vi "Start.vi"(11 "Core Actor in":refnum<class "Core Actor.lvclass">) -> (3 "Core Actor out":refnum<class "Core Actor.lvclass">)   [LabVIEW 2025, in "jettl.lvlib" / "Core Actor.lvlib" / "Core Actor.lvclass"]
uses:
  Core Actor.lvclass
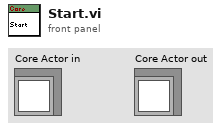
[diagram p1: front panel]
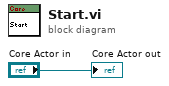
[diagram p0: block diagram]
diagram:
  "Core Actor out" <- "Core Actor in"
